vi "GetType.vi"(8 "error in (no error)":errorcluster, 11 "Set Lengths Msg":refnum<class "Set Lengths Msg.lvclass">) -> (0 "error out":errorcluster, 2 "Data Sample":variant, 3 "Set Lengths Msg":refnum<class "Set Lengths Msg.lvclass">)   [LabVIEW 2021, in "BNT_ULx.lvlib" / "Set Lengths Msg.lvclass"]
uses:
  Set Lengths Msg.lvclass
  Set Lengths Msg.lvclass/Set Lengths Msg.ctl
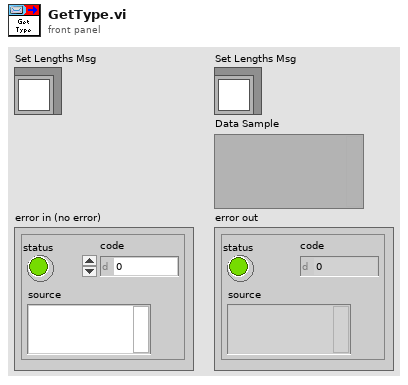
[diagram p1: front panel]
types:
  T1 = cluster{"PWM Lengths":dbl[unit][], "Start Index":i32}
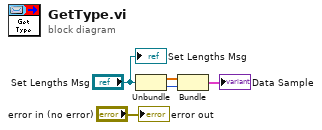
[diagram p0: block diagram]
diagram:
  n1 = Unbundle("Set Lengths Msg") -> (w2:dbl[unit][], w1:i32)
  n2 = Bundle("PWM Lengths"=w2, "Start Index"=w1) -> (→"Data Sample":T1)  [unwired: 1 in]
  "error out" <- "error in (no error)"
  "Set Lengths Msg" <- "Set Lengths Msg"
